vi "Run.vi"(8 "error in (no error)":errorcluster, 11 "Channel in":refnum<class "Channel.lvclass">) -> (0 "error out":errorcluster, 3 "Channel out":refnum<class "Channel.lvclass">)   [LabVIEW 2018, in "Channel.lvclass"]
doc: "Run the channel"
uses:
  Channel.lvclass
  Channel.lvclass/Channel.ctl
  Simulated_CCD_Camera/Simulated_CCD_Camera.lvclass/Simulated_CCD_Camera.ctl
  State Machine/State Machine.lvclass
  Simulated_CCD_Camera/Simulated_CCD_Camera.lvclass
  RxTx/RxTx.lvclass
  Header content/Header content.lvclass
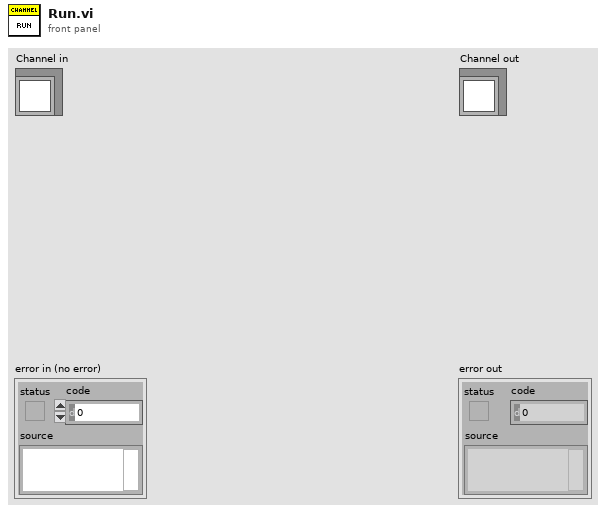
[diagram p1: front panel]
types:
  T1 = cluster{"PREAMP":u16, "READOUT_RATE":u16, "EM_GAIN":u16, "VERTICAL_SHIFT_SPEED":u16, "READ_MODE":u16, "FRAME_TRANSFER":bool, "VERTICAL_CLOCK_VOLTAGE":u16, "ACQUISITION_MODE":u16, "AD_CHANNEL":u16, "EM_MODE":u16, "SHUTTER_TTL":u16, "SHUTTER_OPENING_TIME":u16, "SHUTTER_CLOSING_TIME":u16, "SHUTTER_MODE":u16, "TRIGGER_MODE":u16, "VBIN":u16, "INITIAL_LINE":u16, "INITIAL_COLUMN":u16, "FINAL_LINE":u16, "FINAL_COLUMN":u16, "HBIN":u16}
  T2 = cluster{"CYCLES_DONE":u16, "LAST_IMAGE_NAME":string, "DISK_SPACE":u16, "FRAMES_DONE":u16, "CCD_STATUS":string, "CURRENT_TEMPERATURE":i16, "TEMPERATURE_STATUS":string, "FRAME_EXPOSURE_TIME":sgl, "ERROR":bool, "SERIAL_NUMBER":u16, "ACQUIRING":bool, "IMAGE_INDEX":u32, "SEQS_DONE":u16}
  T3 = cluster{"COOLER_POWER_STATUS":u16, "TEMP":i32, "EXPTIME":dbl, "#FRAMES":u32, "#CYCLES":u32, "COMMENT":string, "OBSTYPE":string, "OBJECT":string, "OBSERVER":string, "FILTER":string, "CTRLINTE":string, "INSTMODE":string, "#SEQS":u32, "WAVEPLATE_POS":u16, "TCSMODE":bool, "INSTROT":dbl, "ICSMODE":u8}
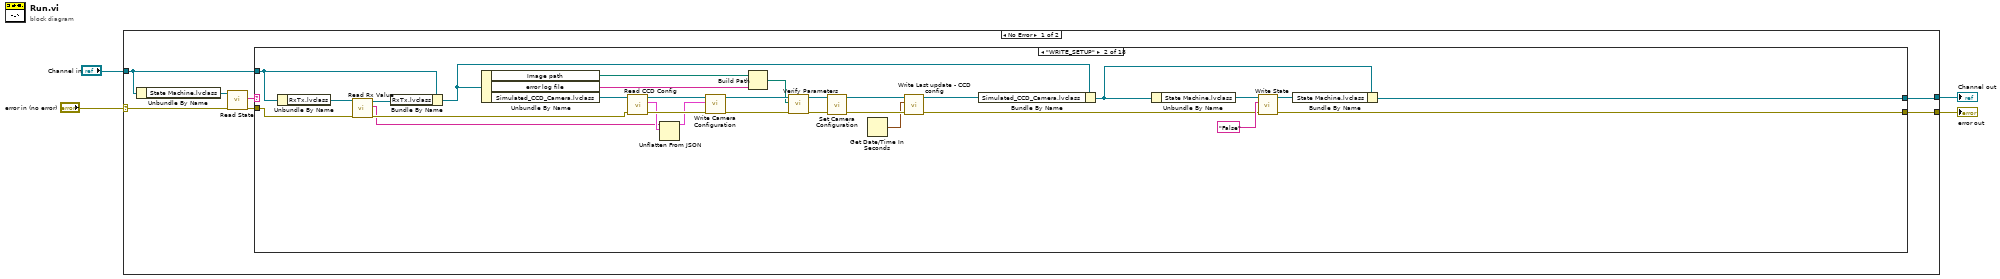
[diagram p0: block diagram]
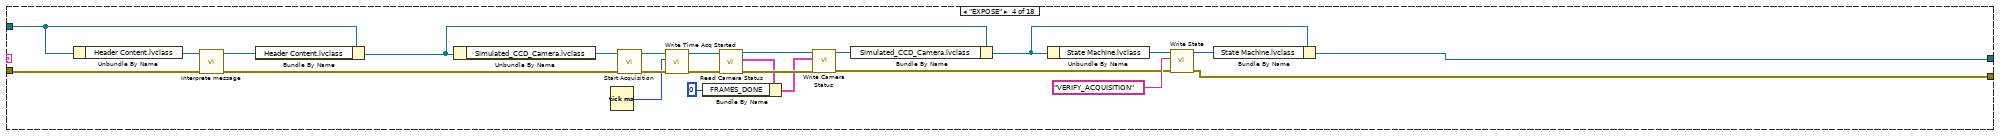
[diagram p4: hidden frame]
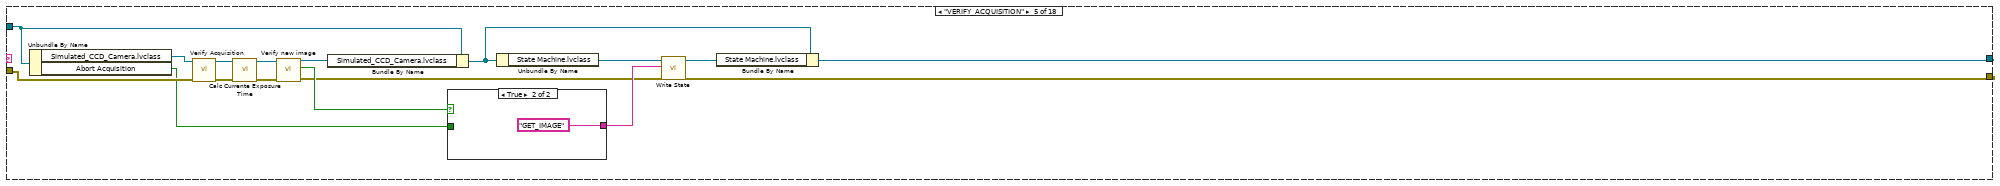
[diagram p5: hidden frame]
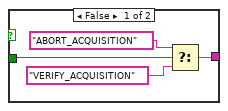
[diagram p6: hidden frame]
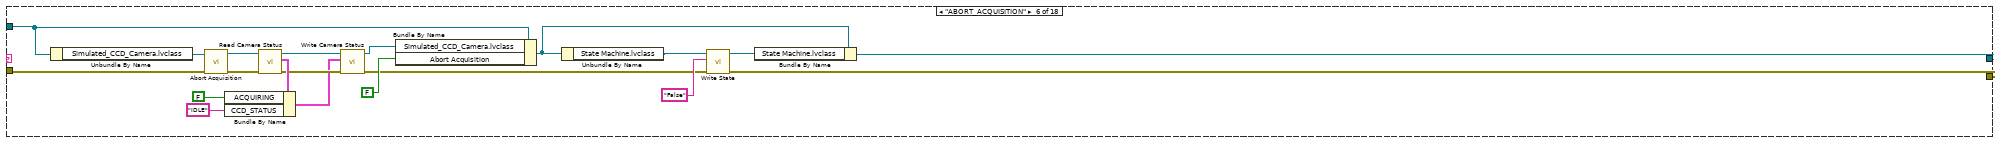
[diagram p7: hidden frame]
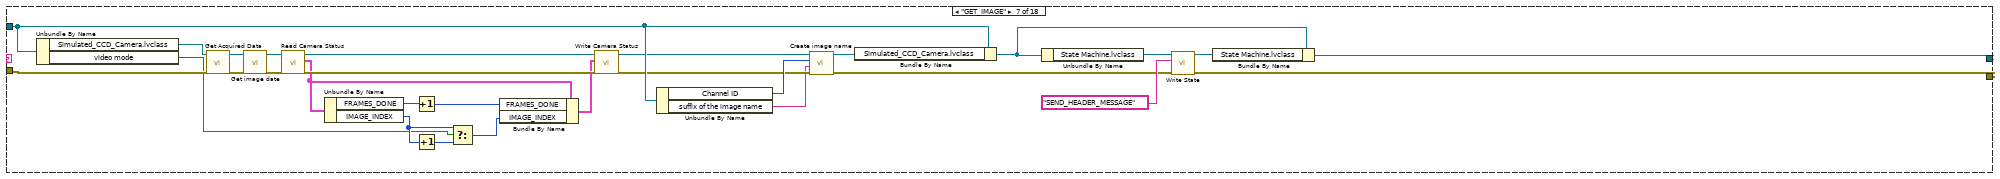
[diagram p8: hidden frame]
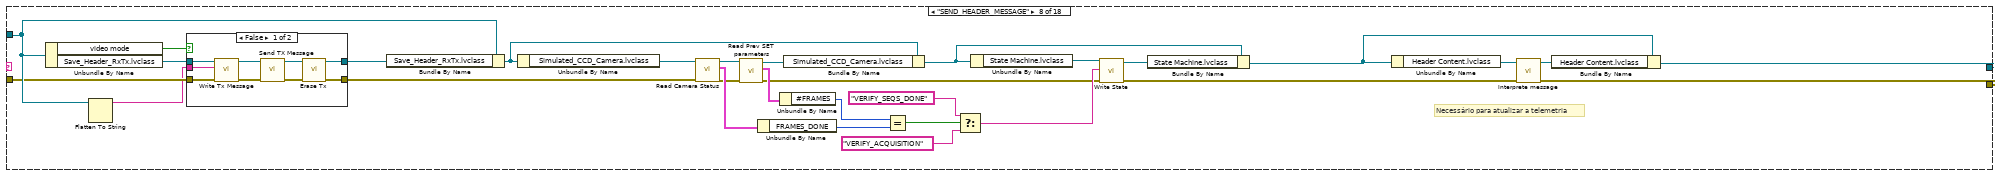
[diagram p9: hidden frame]
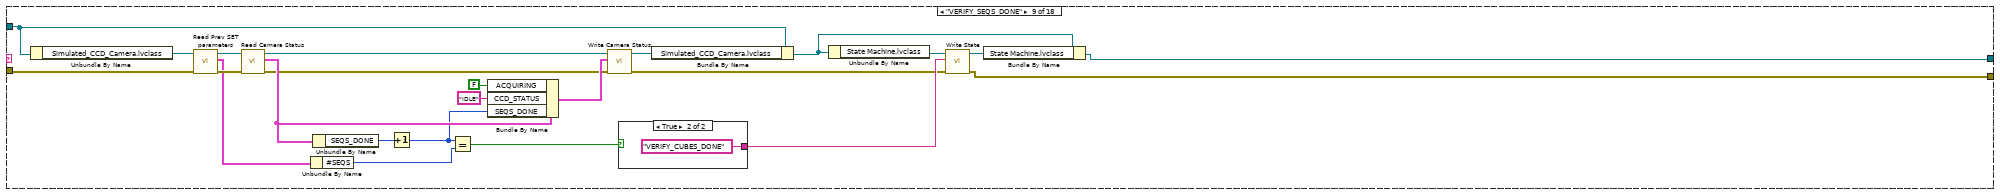
[diagram p11: hidden frame]
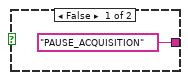
[diagram p12: hidden frame]
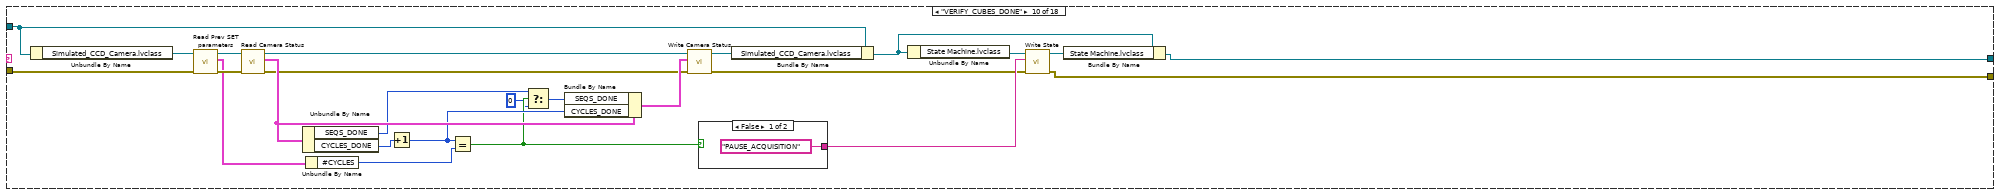
[diagram p13: hidden frame]
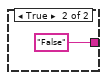
[diagram p14: hidden frame]
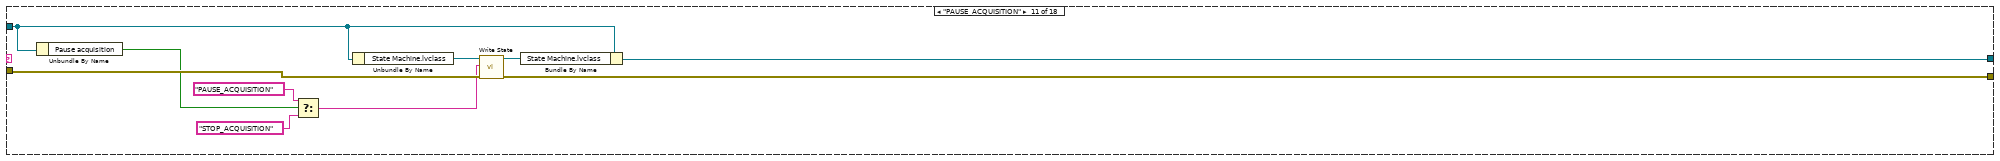
[diagram p15: hidden frame]
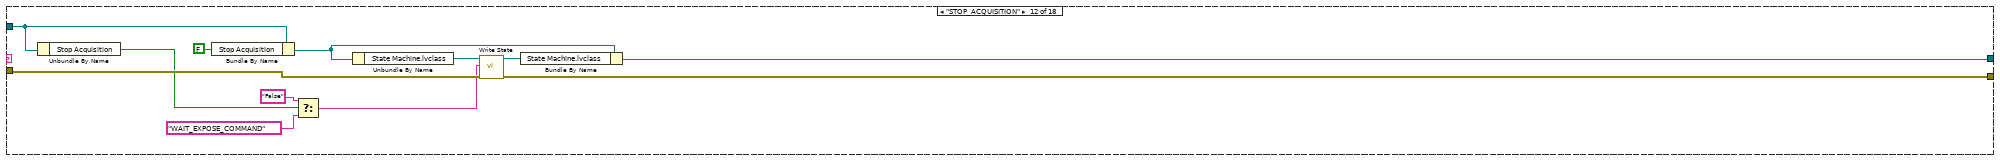
[diagram p16: hidden frame]
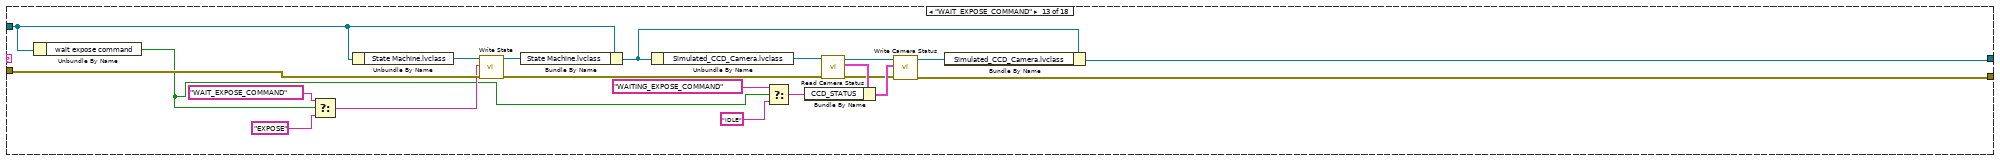
[diagram p17: hidden frame]
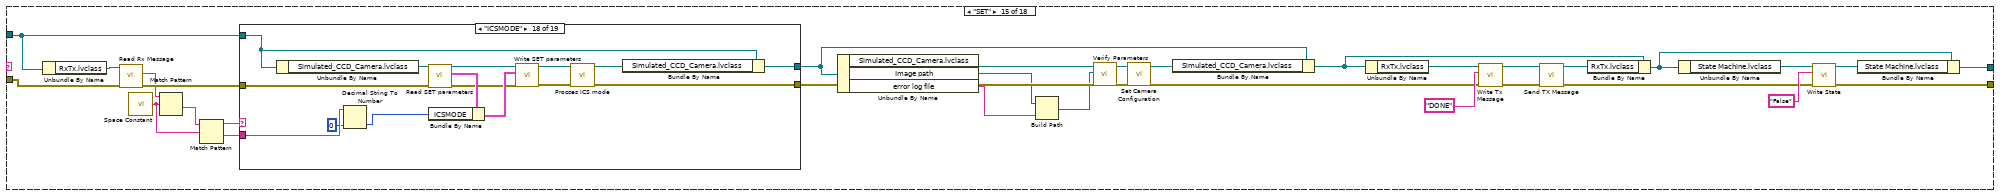
[diagram p19: hidden frame]
diagram:
  n1 = case shown="No Error" "error in (no error)" {
    selector: "error in (no error)" -> [w7 w618]
    tunnel: [w11 w618] -> w3
    tunnel: [w9 w617] -> w1
    tunnel: "Channel in" -> [w10 w617]
    frame No Error {
      n2 = Unbundle By Name(w10) -> ("State Machine.lvclass"=w8:refnum<class "State Machine.lvclass">)
      n3 = call-dynamic "Read State.vi"("error in (no error)"=w7, "State Machine in"=w8) -> ("error out"=w6:errorcluster, "State"=w5:string)  [unwired: 7 in, 1 out]
      n4 = case shown="\"WRITE_SETUP\"" w5 {
        tunnel: w6 -> [w12 w35 w44 w50 w75 w97 w136 w152 w193 w221 w243 w254 w276 w279 w302 w544 w604 w613]
        tunnel: [w12 w38 w44 w66 w82 w108 w138 w142 w187 w215 w241 w252 w262 w279 w304 w537 w595 w605] -> w11
        tunnel: [w13 w39 w45 w65 w85 w111 w119 w143 w188 w216 w240 w251 w263 w280 w305 w538 w602 w606] -> w9
        tunnel: w10 -> [w13 w42 w45 w49 w87 w96 w128 w154 w198 w228 w242 w253 w275 w280 w311 w535 w603 w610]
        frame "False", Default {
        }
        frame "WRITE_SETUP" {
          n5 = Unbundle By Name(w42) -> ("RxTx.lvclass"=w36:refnum<class "RxTx.lvclass">)
          n6 = call "Read Rx Value.vi"("error in (no error)"=w35, "RxTx in"=w36) -> ("error out"=w30:errorcluster, "Rx value"=w27:string, "RxTx out"=w34:refnum<class "RxTx.lvclass">)  [unwired: 7 in]
          n7 = Bundle By Name(cluster=w42, "RxTx.lvclass"=w34) -> (w43:refnum<class "Channel.lvclass">)
          n8 = Unbundle By Name(w43) -> ("Image path"=w14:path, "error log file"=w15:string, "Simulated_CCD_Camera.lvclass"=w33:refnum<class "Simulated_CCD_Camera.lvclass">)
          n9 = call "Read CCD Config.vi"("error in (no error)"=w30, "CCDCamera in"=w33) -> ("error out"=w31:errorcluster, "CCD Config"=w29:T1, "CCDCamera out"=w32:refnum<class "Simulated_CCD_Camera.lvclass">)  [unwired: 7 in]
          n10 = Unflatten From JSON(JSON string=w27, type and defaults=w29) -> (value=w28:T1)  [unwired: 5 in, 1 out]
          n11 = call-dynamic "Write Camera Configuration.vi"("error in (no error)"=w31, "CCD Config"=w28, "CCDCamera in"=w32) -> ("error out"=w25:errorcluster, "CCDCamera out"=w24:refnum<class "Simulated_CCD_Camera.lvclass">)  [unwired: 7 in]
          n12 = Build Path(base path=w14, name or relative path=w15) -> (appended path=w16:path)
          n13 = call "Verify Parameters.vi"("error in (no error)"=w25, "error file"=w16, "Simulated_CCD_Camera in"=w24) -> ("error out"=w23:errorcluster, "Simulated_CCD_Camera out"=w22:refnum<class "Simulated_CCD_Camera.lvclass">)  [unwired: 7 in]
          n14 = call-dynamic "Set Camera Configuration.vi"("error in (no error)"=w23, "CCDCamera in"=w22) -> ("error out"=w19:errorcluster, "CCDCamera out"=w21:refnum<class "Simulated_CCD_Camera.lvclass">)  [unwired: 8 in]
          n15 = Get Date/Time In Seconds() -> (seconds since 1Jan1904=w17:timestamp)
          n16 = call-dynamic "Write Last update - CCD config.vi"("error in (no error)"=w19, "Last update - CCD config"=w17, "Simulated_CCD_Camera in"=w21) -> ("error out"=w18:errorcluster, "Simulated_CCD_Camera out"=w20:refnum<class "Simulated_CCD_Camera.lvclass">)  [unwired: 7 in]
          n17 = Bundle By Name(cluster=w43, "Simulated_CCD_Camera.lvclass"=w20) -> (w37:refnum<class "Channel.lvclass">)
          n18 = Unbundle By Name(w37) -> ("State Machine.lvclass"=w40:refnum<class "State Machine.lvclass">)
          n19 = call-dynamic "Write State.vi"("error in (no error)"=w18, "State"="False", "State Machine in"=w40) -> ("error out"=w38:errorcluster, "State Machine out"=w41:refnum<class "State Machine.lvclass">)  [unwired: 7 in]
          n20 = Bundle By Name(cluster=w37, "State Machine.lvclass"=w41) -> (w39:refnum<class "Channel.lvclass">)
        }
        frame "---------------------------------" {
        }
        frame "EXPOSE" {
          n21 = Unbundle By Name(w49) -> ("Header Content.lvclass"=w51:refnum<class "Header content.lvclass">)
          n22 = call "Interprete message.vi"("error in (no error)"=w50, "TCS_ACS in"=w51) -> ("error out"=w47:errorcluster, "TCS_ACS out"=w48:refnum<class "Header content.lvclass">)  [unwired: 8 in]
          n23 = Bundle By Name(cluster=w49, "Header Content.lvclass"=w48) -> (w46:refnum<class "Channel.lvclass">)
          n24 = Unbundle By Name(w46) -> ("Simulated_CCD_Camera.lvclass"=w68:refnum<class "Simulated_CCD_Camera.lvclass">)
          n25 = Tick Count (ms)() -> (millisecond timer value=w61:u32)
          n26 = call-dynamic "Start Acquisition.vi"("error in (no error)"=w47, "CCDCamera in"=w68) -> ("error out"=w62:errorcluster, "CCDCamera out"=w63:refnum<class "Simulated_CCD_Camera.lvclass">)  [unwired: 8 in]
          n27 = call "Write Time Acq Started.vi"("error in (no error)"=w62, "Time Acq Started"=w61, "Simulated_CCD_Camera in"=w63) -> ("error out"=w57:errorcluster, "Simulated_CCD_Camera out"=w58:refnum<class "Simulated_CCD_Camera.lvclass">)  [unwired: 7 in]
          n28 = call "Read Camera Status.vi"("error in (no error)"=w57, "CCDCamera in"=w58) -> ("error out"=w56:errorcluster, "Camera Status"=w54:T2, "CCDCamera out"=w55:refnum<class "Simulated_CCD_Camera.lvclass">)  [unwired: 7 in]
          n29 = Bundle By Name(cluster=w54, "FRAMES_DONE"=u16 0) -> (w53:T2)
          n30 = call "Write Camera Status.vi"("error in (no error)"=w56, "Camera Status"=w53, "CCDCamera in"=w55) -> ("error out"=w59:errorcluster, "CCDCamera out"=w60:refnum<class "Simulated_CCD_Camera.lvclass">)  [unwired: 7 in]
          n31 = Bundle By Name(cluster=w46, "Simulated_CCD_Camera.lvclass"=w60) -> (w64:refnum<class "Channel.lvclass">)
          n32 = Unbundle By Name(w64) -> ("State Machine.lvclass"=w70:refnum<class "State Machine.lvclass">)
          n33 = call-dynamic "Write State.vi"("error in (no error)"=w59, "State"="VERIFY_ACQUISITION", "State Machine in"=w70) -> ("error out"=w66:errorcluster, "State Machine out"=w67:refnum<class "State Machine.lvclass">)  [unwired: 7 in]
          n34 = Bundle By Name(cluster=w64, "State Machine.lvclass"=w67) -> (w65:refnum<class "Channel.lvclass">)
        }
        frame "VERIFY_ACQUISITION" {
          n35 = Unbundle By Name(w87) -> ("Simulated_CCD_Camera.lvclass"=w76:refnum<class "Simulated_CCD_Camera.lvclass">, "Abort Acquisition"=w74:bool)
          n36 = call-dynamic "Verify Acquisition.vi"("error in (no error)"=w75, "CCDCamera in"=w76) -> ("error out"=w78:errorcluster, "CCDCamera out"=w73:refnum<class "Simulated_CCD_Camera.lvclass">)  [unwired: 8 in]
          n37 = call-dynamic "Calc Currente Exposure Time.vi"("error in (no error)"=w78, "CCDCamera in"=w73) -> ("error out"=w79:errorcluster, "CCDCamera out"=w71:refnum<class "Simulated_CCD_Camera.lvclass">)  [unwired: 8 in]
          n38 = call-dynamic "Verify new image.vi"("error in (no error)"=w79, "CCDCamera in"=w71) -> ("error out"=w77:errorcluster, "New Images ?"=w80:bool, "CCDCamera out"=w72:refnum<class "Simulated_CCD_Camera.lvclass">)  [unwired: 7 in]
          n39 = Bundle By Name(cluster=w87, "Simulated_CCD_Camera.lvclass"=w72) -> (w86:refnum<class "Channel.lvclass">)
          n40 = case shown="True" w80 {
            tunnel: [w89 "GET_IMAGE"] -> w81
            tunnel: w74 -> [w88 _]
            frame False {
              n41 = Select(t="ABORT_ACQUISITION", s=w88, f="VERIFY_ACQUISITION") -> (s? t:f=w89:string)
            }
            frame True {
            }
          }
          n42 = Unbundle By Name(w86) -> ("State Machine.lvclass"=w84:refnum<class "State Machine.lvclass">)
          n43 = call-dynamic "Write State.vi"("error in (no error)"=w77, "State"=w81, "State Machine in"=w84) -> ("error out"=w82:errorcluster, "State Machine out"=w83:refnum<class "State Machine.lvclass">)  [unwired: 7 in]
          n44 = Bundle By Name(cluster=w86, "State Machine.lvclass"=w83) -> (w85:refnum<class "Channel.lvclass">)
        }
        frame "ABORT_ACQUISITION" {
          n45 = Unbundle By Name(w96) -> ("Simulated_CCD_Camera.lvclass"=w98:refnum<class "Simulated_CCD_Camera.lvclass">)
          n46 = call-dynamic "Abort Acquisition.vi"("error in (no error)"=w97, "CCDCamera in"=w98) -> ("error out"=w103:errorcluster, "CCDCamera out"=w104:refnum<class "Simulated_CCD_Camera.lvclass">)  [unwired: 8 in]
          n47 = call "Read Camera Status.vi"("error in (no error)"=w103, "CCDCamera in"=w104) -> ("error out"=w101:errorcluster, "Camera Status"=w106:T2, "CCDCamera out"=w102:refnum<class "Simulated_CCD_Camera.lvclass">)  [unwired: 7 in]
          n48 = Bundle By Name(cluster=w106, "ACQUIRING"=FALSE ("Acquiring"), "CCD_STATUS"="IDLE" ("STATUS")) -> (w100:T2)
          n49 = call "Write Camera Status.vi"("error in (no error)"=w101, "Camera Status"=w100, "CCDCamera in"=w102) -> ("error out"=w94:errorcluster, "CCDCamera out"=w93:refnum<class "Simulated_CCD_Camera.lvclass">)  [unwired: 7 in]
          n50 = Bundle By Name(cluster=w96, "Simulated_CCD_Camera.lvclass"=w93, "Abort Acquisition"=FALSE ("Acquiring")) -> (w112:refnum<class "Channel.lvclass">)
          n51 = Unbundle By Name(w112) -> ("State Machine.lvclass"=w110:refnum<class "State Machine.lvclass">)
          n52 = call-dynamic "Write State.vi"("error in (no error)"=w94, "State"="False", "State Machine in"=w110) -> ("error out"=w108:errorcluster, "State Machine out"=w109:refnum<class "State Machine.lvclass">)  [unwired: 7 in]
          n53 = Bundle By Name(cluster=w112, "State Machine.lvclass"=w109) -> (w111:refnum<class "Channel.lvclass">)
        }
        frame "GET_IMAGE" {
          n54 = Unbundle By Name(w128) -> ("Simulated_CCD_Camera.lvclass"=w116:refnum<class "Simulated_CCD_Camera.lvclass">, "video mode"=w113:bool)
          n55 = call-dynamic "Get Acquired Data.vi"("error in (no error)"=w136, "CCDCamera in"=w116) -> ("error out"=w120:errorcluster, "CCDCamera out"=w123:refnum<class "Simulated_CCD_Camera.lvclass">)  [unwired: 8 in]
          n56 = call-dynamic "Get image date.vi"("error in (no error)"=w120, "Simulated_CCD_Camera in"=w123) -> ("error out"=w121:errorcluster, "Simulated_CCD_Camera out"=w122:refnum<class "Simulated_CCD_Camera.lvclass">)  [unwired: 8 in]
          n57 = call "Read Camera Status.vi"("error in (no error)"=w121, "CCDCamera in"=w122) -> ("error out"=w135:errorcluster, "Camera Status"=w131:T2, "CCDCamera out"=w134:refnum<class "Simulated_CCD_Camera.lvclass">)  [unwired: 7 in]
          n58 = Unbundle By Name(w131) -> ("FRAMES_DONE"=w133:u16, "IMAGE_INDEX"=w114:u32)
          n59 = Increment(x=w133) -> (x+1=w117:u16)
          n60 = Increment(x=w114) -> (x+1=w115:u32)
          n61 = Select(t=w114, s=w113, f=w115) -> (s? t:f=w118:u32)
          n62 = Bundle By Name(cluster=w131, "FRAMES_DONE"=w117, "IMAGE_INDEX"=w118) -> (w132:T2)
          n63 = call "Write Camera Status.vi"("error in (no error)"=w135, "Camera Status"=w132, "CCDCamera in"=w134) -> ("error out"=w125:errorcluster, "CCDCamera out"=w126:refnum<class "Simulated_CCD_Camera.lvclass">)  [unwired: 7 in]
          n64 = Unbundle By Name(w128) -> ("Channel ID"=w127:u8, "suffix of the image name"=w124:string)
          n65 = call "Create image name.vi"("error in (no error)"=w125, "Suffix"=w124, "Channel"=w127, "Simulated_CCD_Camera in"=w126) -> ("error out"=w129:errorcluster, "Simulated_CCD_Camera out"=w130:refnum<class "Simulated_CCD_Camera.lvclass">)  [unwired: 6 in]
          n66 = Bundle By Name(cluster=w128, "Simulated_CCD_Camera.lvclass"=w130) -> (w141:refnum<class "Channel.lvclass">)
          n67 = Unbundle By Name(w141) -> ("State Machine.lvclass"=w139:refnum<class "State Machine.lvclass">)
          n68 = call-dynamic "Write State.vi"("error in (no error)"=w129, "State"="SEND_HEADER_MESSAGE", "State Machine in"=w139) -> ("error out"=w138:errorcluster, "State Machine out"=w140:refnum<class "State Machine.lvclass">)  [unwired: 7 in]
          n69 = Bundle By Name(cluster=w141, "State Machine.lvclass"=w140) -> (w119:refnum<class "Channel.lvclass">)
        }
        frame "SEND_HEADER_MESSAGE" {
          # "Necessário para atualizar a telemetria"
          n70 = Unbundle By Name(w154) -> ("video mode"=w148:bool, "Save_Header_RxTx.lvclass"=w153:refnum<class "RxTx.lvclass">)
          n71 = Flatten To String(anything=w154) -> (data string=w149:string)  [unwired: 3 in, 2 out]
          n72 = case shown="False" w148 {
            tunnel: w153 -> [w180 w182]
            tunnel: w152 -> [w177 w181]
            tunnel: [w175 w182] -> w151
            tunnel: [w173 w181] -> w150
            tunnel: w149 -> [w172 _]
            frame False {
              n73 = call "Write Tx Message.vi"("error in (no error)"=w177, "Tx Message"=w172, "RxTx in"=w180) -> ("error out"=w178:errorcluster, "RxTx out"=w179:refnum<class "RxTx.lvclass">)  [unwired: 7 in]
              n74 = call "Send TX Message.vi"("error in (no error)"=w178, "RxTx in"=w179) -> ("error out"=w174:errorcluster, "RxTx out"=w176:refnum<class "RxTx.lvclass">)  [unwired: 8 in]
              n75 = call "Erase Tx.vi"("error in (no error)"=w174, "RxTx in"=w176) -> ("error out"=w173:errorcluster, "RxTx out"=w175:refnum<class "RxTx.lvclass">)  [unwired: 8 in]
            }
            frame True {
            }
          }
          n76 = Bundle By Name(cluster=w154, "Save_Header_RxTx.lvclass"=w151) -> (w167:refnum<class "Channel.lvclass">)
          n77 = Unbundle By Name(w167) -> ("Simulated_CCD_Camera.lvclass"=w162:refnum<class "Simulated_CCD_Camera.lvclass">)
          n78 = call "Read Camera Status.vi"("error in (no error)"=w150, "CCDCamera in"=w162) -> ("error out"=w158:errorcluster, "Camera Status"=w161:T2, "CCDCamera out"=w160:refnum<class "Simulated_CCD_Camera.lvclass">)  [unwired: 7 in]
          n79 = call-dynamic "Read Prev SET parameters.vi"("error in (no error)"=w158, "Simulated_CCD_Camera in"=w160) -> ("error out"=w155:errorcluster, "Old SET parameters"=w157:T3, "Simulated_CCD_Camera out"=w159:refnum<class "Simulated_CCD_Camera.lvclass">)  [unwired: 7 in]
          n80 = Unbundle By Name(w161) -> ("FRAMES_DONE"=w169:u16)
          n81 = Unbundle By Name(w157) -> ("#FRAMES"=w156:u32)
          n82 = Bundle By Name(cluster=w167, "Simulated_CCD_Camera.lvclass"=w159) -> (w165:refnum<class "Channel.lvclass">)
          n83 = Equal?(x=w156, y=w169) -> (x = y?=w168:bool)
          n84 = Select(t="VERIFY_SEQS_DONE", s=w168, f="VERIFY_ACQUISITION") -> (s? t:f=w166:string)
          n85 = Unbundle By Name(w165) -> ("State Machine.lvclass"=w170:refnum<class "State Machine.lvclass">)
          n86 = call-dynamic "Write State.vi"("error in (no error)"=w155, "State"=w166, "State Machine in"=w170) -> ("error out"=w144:errorcluster, "State Machine out"=w171:refnum<class "State Machine.lvclass">)  [unwired: 7 in]
          n87 = Bundle By Name(cluster=w165, "State Machine.lvclass"=w171) -> (w145:refnum<class "Channel.lvclass">)
          n88 = Unbundle By Name(w145) -> ("Header Content.lvclass"=w147:refnum<class "Header content.lvclass">)
          n89 = call "Interprete message.vi"("error in (no error)"=w144, "TCS_ACS in"=w147) -> ("error out"=w142:errorcluster, "TCS_ACS out"=w146:refnum<class "Header content.lvclass">)  [unwired: 8 in]
          n90 = Bundle By Name(cluster=w145, "Header Content.lvclass"=w146) -> (w143:refnum<class "Channel.lvclass">)
        }
        frame "VERIFY_SEQS_DONE" {
          n91 = Unbundle By Name(w198) -> ("Simulated_CCD_Camera.lvclass"=w196:refnum<class "Simulated_CCD_Camera.lvclass">)
          n92 = call-dynamic "Read Prev SET parameters.vi"("error in (no error)"=w193, "Simulated_CCD_Camera in"=w196) -> ("error out"=w194:errorcluster, "Old SET parameters"=w192:T3, "Simulated_CCD_Camera out"=w195:refnum<class "Simulated_CCD_Camera.lvclass">)  [unwired: 7 in]
          n93 = call "Read Camera Status.vi"("error in (no error)"=w194, "CCDCamera in"=w195) -> ("error out"=w185:errorcluster, "Camera Status"=w204:T2, "CCDCamera out"=w186:refnum<class "Simulated_CCD_Camera.lvclass">)  [unwired: 7 in]
          n94 = Unbundle By Name(w192) -> ("#SEQS"=w191:u32)
          n95 = Unbundle By Name(w204) -> ("SEQS_DONE"=w203:u16)
          n96 = Increment(x=w203) -> (x+1=w201:u16)
          n97 = Equal?(x=w201, y=w191) -> (x = y?=w199:bool)
          n98 = Bundle By Name(cluster=w204, "ACQUIRING"=FALSE, "CCD_STATUS"="IDLE", "SEQS_DONE"=w201) -> (w202:T2)
          n99 = call "Write Camera Status.vi"("error in (no error)"=w185, "Camera Status"=w202, "CCDCamera in"=w186) -> ("error out"=w189:errorcluster, "CCDCamera out"=w190:refnum<class "Simulated_CCD_Camera.lvclass">)  [unwired: 7 in]
          n100 = case shown="True" w199 {
            tunnel: ["PAUSE_ACQUISITION" "VERIFY_CUBES_DONE"] -> w205
            frame False {
            }
            frame True {
            }
          }
          n101 = Bundle By Name(cluster=w198, "Simulated_CCD_Camera.lvclass"=w190) -> (w197:refnum<class "Channel.lvclass">)
          n102 = Unbundle By Name(w197) -> ("State Machine.lvclass"=w200:refnum<class "State Machine.lvclass">)
          n103 = call-dynamic "Write State.vi"("error in (no error)"=w189, "State"=w205, "State Machine in"=w200) -> ("error out"=w187:errorcluster, "State Machine out"=w206:refnum<class "State Machine.lvclass">)  [unwired: 7 in]
          n104 = Bundle By Name(cluster=w197, "State Machine.lvclass"=w206) -> (w188:refnum<class "Channel.lvclass">)
        }
        frame "VERIFY_CUBES_DONE" {
          n105 = Unbundle By Name(w228) -> ("Simulated_CCD_Camera.lvclass"=w224:refnum<class "Simulated_CCD_Camera.lvclass">)
          n106 = call-dynamic "Read Prev SET parameters.vi"("error in (no error)"=w221, "Simulated_CCD_Camera in"=w224) -> ("error out"=w222:errorcluster, "Old SET parameters"=w220:T3, "Simulated_CCD_Camera out"=w223:refnum<class "Simulated_CCD_Camera.lvclass">)  [unwired: 7 in]
          n107 = call "Read Camera Status.vi"("error in (no error)"=w222, "CCDCamera in"=w223) -> ("error out"=w225:errorcluster, "Camera Status"=w231:T2, "CCDCamera out"=w226:refnum<class "Simulated_CCD_Camera.lvclass">)  [unwired: 7 in]
          n108 = Unbundle By Name(w231) -> ("SEQS_DONE"=w210:u16, "CYCLES_DONE"=w209:u16)
          n109 = Unbundle By Name(w220) -> ("#CYCLES"=w219:u32)
          n110 = Increment(x=w209) -> (x+1=w214:u16)
          n111 = Equal?(x=w214, y=w219) -> (x = y?=w212:bool)
          n112 = Select(t=w210, s=w212, f=0) -> (s? t:f=w213:i32)
          n113 = Bundle By Name(cluster=w231, "SEQS_DONE"=w213, "CYCLES_DONE"=w214) -> (w230:T2)
          n114 = call "Write Camera Status.vi"("error in (no error)"=w225, "Camera Status"=w230, "CCDCamera in"=w226) -> ("error out"=w217:errorcluster, "CCDCamera out"=w218:refnum<class "Simulated_CCD_Camera.lvclass">)  [unwired: 7 in]
          n115 = case shown="False" w212 {
            tunnel: ["PAUSE_ACQUISITION" "False"] -> w232
            frame False {
            }
            frame True {
            }
          }
          n116 = Bundle By Name(cluster=w228, "Simulated_CCD_Camera.lvclass"=w218) -> (w227:refnum<class "Channel.lvclass">)
          n117 = Unbundle By Name(w227) -> ("State Machine.lvclass"=w229:refnum<class "State Machine.lvclass">)
          n118 = call-dynamic "Write State.vi"("error in (no error)"=w217, "State"=w232, "State Machine in"=w229) -> ("error out"=w215:errorcluster, "State Machine out"=w233:refnum<class "State Machine.lvclass">)  [unwired: 7 in]
          n119 = Bundle By Name(cluster=w227, "State Machine.lvclass"=w233) -> (w216:refnum<class "Channel.lvclass">)
        }
        frame "PAUSE_ACQUISITION" {
          n120 = Unbundle By Name(w242) -> ("Pause acquisition"=w238:bool)
          n121 = Select(t="PAUSE_ACQUISITION", s=w238, f="STOP_ACQUISITION") -> (s? t:f=w239:string)
          n122 = Unbundle By Name(w242) -> ("State Machine.lvclass"=w245:refnum<class "State Machine.lvclass">)
          n123 = call-dynamic "Write State.vi"("error in (no error)"=w243, "State"=w239, "State Machine in"=w245) -> ("error out"=w241:errorcluster, "State Machine out"=w244:refnum<class "State Machine.lvclass">)  [unwired: 7 in]
          n124 = Bundle By Name(cluster=w242, "State Machine.lvclass"=w244) -> (w240:refnum<class "Channel.lvclass">)
        }
        frame "STOP_ACQUISITION" {
          n125 = Unbundle By Name(w253) -> ("Stop Acquisition"=w246:bool)
          n126 = Bundle By Name(cluster=w253, "Stop Acquisition"=FALSE) -> (w255:refnum<class "Channel.lvclass">)
          n127 = Select(t="False", s=w246, f="WAIT_EXPOSE_COMMAND") -> (s? t:f=w248:string)
          n128 = Unbundle By Name(w255) -> ("State Machine.lvclass"=w257:refnum<class "State Machine.lvclass">)
          n129 = call-dynamic "Write State.vi"("error in (no error)"=w254, "State"=w248, "State Machine in"=w257) -> ("error out"=w252:errorcluster, "State Machine out"=w256:refnum<class "State Machine.lvclass">)  [unwired: 7 in]
          n130 = Bundle By Name(cluster=w255, "State Machine.lvclass"=w256) -> (w251:refnum<class "Channel.lvclass">)
        }
        frame "WAIT_EXPOSE_COMMAND" {
          n131 = Unbundle By Name(w275) -> ("wait expose command"=w258:bool)
          n132 = Select(t="WAIT_EXPOSE_COMMAND", s=w258, f="EXPOSE") -> (s? t:f=w272:string)
          n133 = Unbundle By Name(w275) -> ("State Machine.lvclass"=w278:refnum<class "State Machine.lvclass">)
          n134 = call-dynamic "Write State.vi"("error in (no error)"=w276, "State"=w272, "State Machine in"=w278) -> ("error out"=w270:errorcluster, "State Machine out"=w277:refnum<class "State Machine.lvclass">)  [unwired: 7 in]
          n135 = Bundle By Name(cluster=w275, "State Machine.lvclass"=w277) -> (w265:refnum<class "Channel.lvclass">)
          n136 = Unbundle By Name(w265) -> ("Simulated_CCD_Camera.lvclass"=w271:refnum<class "Simulated_CCD_Camera.lvclass">)
          n137 = Select(t="WAITING_EXPOSE_COMMAND" ("CCD_STATUS"), s=w258, f="IDLE" ("CCD_STATUS")) -> (s? t:f=w260:string)
          n138 = call "Read Camera Status.vi"("error in (no error)"=w270, "CCDCamera in"=w271) -> ("error out"=w267:errorcluster, "Camera Status"=w269:T2, "CCDCamera out"=w266:refnum<class "Simulated_CCD_Camera.lvclass">)  [unwired: 7 in]
          n139 = Bundle By Name(cluster=w269, "CCD_STATUS"=w260) -> (w268:T2)
          n140 = call "Write Camera Status.vi"("error in (no error)"=w267, "Camera Status"=w268, "CCDCamera in"=w266) -> ("error out"=w262:errorcluster, "CCDCamera out"=w264:refnum<class "Simulated_CCD_Camera.lvclass">)  [unwired: 7 in]
          n141 = Bundle By Name(cluster=w265, "Simulated_CCD_Camera.lvclass"=w264) -> (w263:refnum<class "Channel.lvclass">)
        }
        frame "------------------------------" {
        }
        frame "SET" {
          n142 = Unbundle By Name(w311) -> ("RxTx.lvclass"=w301:refnum<class "RxTx.lvclass">)
          n143 = call "Read Rx Message.vi"("error in (no error)"=w302, "RxTx in"=w301) -> ("error out"=w303:errorcluster, "Rx Message"=w299:string)  [unwired: 7 in, 1 out]
          n144 = call <vilib>:"Space Constant.vi"() -> ("String"=w298:string)
          n145 = Match Pattern(string=w299, regular expression=w298) -> (after substring=w300:string)  [unwired: 1 in, 3 out]
          n146 = Match Pattern(string=w300, regular expression=w298) -> (before substring=w297:string, after substring=w296:string)  [unwired: 1 in, 2 out]
          n147 = case shown="\"ICSMODE\"" w297 {
            tunnel: [w314 w326 w339 w352 w365 w378 w392 w405 w418 w429 w440 w451 w462 w473 w484 w495 w508 w523 w528] -> w291
            tunnel: w311 -> [w314 w327 w340 w353 w366 w379 w393 w406 w419 w430 w441 w452 w463 w474 w485 w496 w509 w524 w529]
            tunnel: [w313 w319 w332 w345 w358 w371 w380 w398 w411 w425 w436 w447 w458 w469 w480 w491 w504 w510 w527] -> w292
            tunnel: w303 -> [w313 w321 w334 w347 w360 w373 w390 w400 w413 w427 w438 w449 w460 w471 w482 w493 w506 w521 w527]
            tunnel: w296 -> [_ w323 w336 w349 w362 w375 w384 w402 w415 w420 w431 w442 w453 w464 w475 w486 w498 w516 w525]
            frame "False", Default {
            }
            frame "EXPTIME" {
              n148 = Unbundle By Name(w327) -> ("Simulated_CCD_Camera.lvclass"=w322:refnum<class "Simulated_CCD_Camera.lvclass">)
              n149 = Fract/Exp String To Number(string=w323, default (0 dbl)=0.0) -> (number=w324:dbl)  [unwired: 2 in, 1 out]
              n150 = call-dynamic "Read SET parameters.vi"("error in (no error)"=w321, "Simulated_CCD_Camera in"=w322) -> ("error out"=w315:errorcluster, "New SET parameters"=w318:T3, "Simulated_CCD_Camera out"=w316:refnum<class "Simulated_CCD_Camera.lvclass">)  [unwired: 7 in]
              n151 = Bundle By Name(cluster=w318, "EXPTIME"=w324) -> (w317:T3)
              n152 = call-dynamic "Write SET parameters.vi"("error in (no error)"=w315, "New SET parameters"=w317, "Simulated_CCD_Camera in"=w316) -> ("error out"=w319:errorcluster, "Simulated_CCD_Camera out"=w320:refnum<class "Simulated_CCD_Camera.lvclass">)  [unwired: 7 in]
              n153 = Bundle By Name(cluster=w327, "Simulated_CCD_Camera.lvclass"=w320) -> (w326:refnum<class "Channel.lvclass">)
            }
            frame "INSTROT" {
              n154 = Unbundle By Name(w340) -> ("Simulated_CCD_Camera.lvclass"=w335:refnum<class "Simulated_CCD_Camera.lvclass">)
              n155 = Fract/Exp String To Number(string=w336, default (0 dbl)=0.0) -> (number=w337:dbl)  [unwired: 2 in, 1 out]
              n156 = call-dynamic "Read SET parameters.vi"("error in (no error)"=w334, "Simulated_CCD_Camera in"=w335) -> ("error out"=w328:errorcluster, "New SET parameters"=w331:T3, "Simulated_CCD_Camera out"=w329:refnum<class "Simulated_CCD_Camera.lvclass">)  [unwired: 7 in]
              n157 = Bundle By Name(cluster=w331, "INSTROT"=w337) -> (w330:T3)
              n158 = call-dynamic "Write SET parameters.vi"("error in (no error)"=w328, "New SET parameters"=w330, "Simulated_CCD_Camera in"=w329) -> ("error out"=w332:errorcluster, "Simulated_CCD_Camera out"=w333:refnum<class "Simulated_CCD_Camera.lvclass">)  [unwired: 7 in]
              n159 = Bundle By Name(cluster=w340, "Simulated_CCD_Camera.lvclass"=w333) -> (w339:refnum<class "Channel.lvclass">)
            }
            frame "#FRAMES" {
              n160 = Unbundle By Name(w353) -> ("Simulated_CCD_Camera.lvclass"=w348:refnum<class "Simulated_CCD_Camera.lvclass">)
              n161 = Fract/Exp String To Number(string=w349, default (0 dbl)=u32 0) -> (number=w350:u32)  [unwired: 2 in, 1 out]
              n162 = call-dynamic "Read SET parameters.vi"("error in (no error)"=w347, "Simulated_CCD_Camera in"=w348) -> ("error out"=w341:errorcluster, "New SET parameters"=w344:T3, "Simulated_CCD_Camera out"=w342:refnum<class "Simulated_CCD_Camera.lvclass">)  [unwired: 7 in]
              n163 = Bundle By Name(cluster=w344, "#FRAMES"=w350) -> (w343:T3)
              n164 = call-dynamic "Write SET parameters.vi"("error in (no error)"=w341, "New SET parameters"=w343, "Simulated_CCD_Camera in"=w342) -> ("error out"=w345:errorcluster, "Simulated_CCD_Camera out"=w346:refnum<class "Simulated_CCD_Camera.lvclass">)  [unwired: 7 in]
              n165 = Bundle By Name(cluster=w353, "Simulated_CCD_Camera.lvclass"=w346) -> (w352:refnum<class "Channel.lvclass">)
            }
            frame "#CYCLES" {
              n166 = Unbundle By Name(w366) -> ("Simulated_CCD_Camera.lvclass"=w361:refnum<class "Simulated_CCD_Camera.lvclass">)
              n167 = Fract/Exp String To Number(string=w362, default (0 dbl)=u32 0) -> (number=w363:u32)  [unwired: 2 in, 1 out]
              n168 = call-dynamic "Read SET parameters.vi"("error in (no error)"=w360, "Simulated_CCD_Camera in"=w361) -> ("error out"=w354:errorcluster, "New SET parameters"=w357:T3, "Simulated_CCD_Camera out"=w355:refnum<class "Simulated_CCD_Camera.lvclass">)  [unwired: 7 in]
              n169 = Bundle By Name(cluster=w357, "#CYCLES"=w363) -> (w356:T3)
              n170 = call-dynamic "Write SET parameters.vi"("error in (no error)"=w354, "New SET parameters"=w356, "Simulated_CCD_Camera in"=w355) -> ("error out"=w358:errorcluster, "Simulated_CCD_Camera out"=w359:refnum<class "Simulated_CCD_Camera.lvclass">)  [unwired: 7 in]
              n171 = Bundle By Name(cluster=w366, "Simulated_CCD_Camera.lvclass"=w359) -> (w365:refnum<class "Channel.lvclass">)
            }
            frame "#SEQS" {
              n172 = Unbundle By Name(w379) -> ("Simulated_CCD_Camera.lvclass"=w374:refnum<class "Simulated_CCD_Camera.lvclass">)
              n173 = Fract/Exp String To Number(string=w375, default (0 dbl)=u32 0) -> (number=w376:u32)  [unwired: 2 in, 1 out]
              n174 = call-dynamic "Read SET parameters.vi"("error in (no error)"=w373, "Simulated_CCD_Camera in"=w374) -> ("error out"=w367:errorcluster, "New SET parameters"=w370:T3, "Simulated_CCD_Camera out"=w368:refnum<class "Simulated_CCD_Camera.lvclass">)  [unwired: 7 in]
              n175 = Bundle By Name(cluster=w370, "#SEQS"=w376) -> (w369:T3)
              n176 = call-dynamic "Write SET parameters.vi"("error in (no error)"=w367, "New SET parameters"=w369, "Simulated_CCD_Camera in"=w368) -> ("error out"=w371:errorcluster, "Simulated_CCD_Camera out"=w372:refnum<class "Simulated_CCD_Camera.lvclass">)  [unwired: 7 in]
              n177 = Bundle By Name(cluster=w379, "Simulated_CCD_Camera.lvclass"=w372) -> (w378:refnum<class "Channel.lvclass">)
            }
            frame "WAVEPLATE_POS" {
              n178 = Unbundle By Name(w393) -> ("Simulated_CCD_Camera.lvclass"=w391:refnum<class "Simulated_CCD_Camera.lvclass">)
              n179 = Decimal String To Number(string=w384) -> (number=w385:i32)  [unwired: 2 in, 1 out]
              n180 = call-dynamic "Read SET parameters.vi"("error in (no error)"=w390, "Simulated_CCD_Camera in"=w391) -> ("error out"=w386:errorcluster, "New SET parameters"=w389:T3, "Simulated_CCD_Camera out"=w387:refnum<class "Simulated_CCD_Camera.lvclass">)  [unwired: 7 in]
              n181 = Bundle By Name(cluster=w389, "WAVEPLATE_POS"=w385) -> (w388:T3)
              n182 = call-dynamic "Write SET parameters.vi"("error in (no error)"=w386, "New SET parameters"=w388, "Simulated_CCD_Camera in"=w387) -> ("error out"=w381:errorcluster, "Simulated_CCD_Camera out"=w383:refnum<class "Simulated_CCD_Camera.lvclass">)  [unwired: 7 in]
              n183 = call "process waveplate string.vi"("error in (no error)"=w381, "Simulated_CCD_Camera in"=w383) -> ("error out"=w380:errorcluster, "Simulated_CCD_Camera out"=w382:refnum<class "Simulated_CCD_Camera.lvclass">)  [unwired: 8 in]
              n184 = Bundle By Name(cluster=w393, "Simulated_CCD_Camera.lvclass"=w382) -> (w392:refnum<class "Channel.lvclass">)
            }
            frame "TEMP" {
              n185 = Unbundle By Name(w406) -> ("Simulated_CCD_Camera.lvclass"=w401:refnum<class "Simulated_CCD_Camera.lvclass">)
              n186 = Fract/Exp String To Number(string=w402, default (0 dbl)=0) -> (number=w403:i32)  [unwired: 2 in, 1 out]
              n187 = call-dynamic "Read SET parameters.vi"("error in (no error)"=w400, "Simulated_CCD_Camera in"=w401) -> ("error out"=w394:errorcluster, "New SET parameters"=w397:T3, "Simulated_CCD_Camera out"=w395:refnum<class "Simulated_CCD_Camera.lvclass">)  [unwired: 7 in]
              n188 = Bundle By Name(cluster=w397, "TEMP"=w403) -> (w396:T3)
              n189 = call-dynamic "Write SET parameters.vi"("error in (no error)"=w394, "New SET parameters"=w396, "Simulated_CCD_Camera in"=w395) -> ("error out"=w398:errorcluster, "Simulated_CCD_Camera out"=w399:refnum<class "Simulated_CCD_Camera.lvclass">)  [unwired: 7 in]
              n190 = Bundle By Name(cluster=w406, "Simulated_CCD_Camera.lvclass"=w399) -> (w405:refnum<class "Channel.lvclass">)
            }
            frame "COOLER_POWER_STATUS" {
              n191 = Unbundle By Name(w419) -> ("Simulated_CCD_Camera.lvclass"=w414:refnum<class "Simulated_CCD_Camera.lvclass">)
              n192 = Fract/Exp String To Number(string=w415, default (0 dbl)=u16 0) -> (number=w416:u16)  [unwired: 2 in, 1 out]
              n193 = call-dynamic "Read SET parameters.vi"("error in (no error)"=w413, "Simulated_CCD_Camera in"=w414) -> ("error out"=w407:errorcluster, "New SET parameters"=w410:T3, "Simulated_CCD_Camera out"=w408:refnum<class "Simulated_CCD_Camera.lvclass">)  [unwired: 7 in]
              n194 = Bundle By Name(cluster=w410, "COOLER_POWER_STATUS"=w416) -> (w409:T3)
              n195 = call-dynamic "Write SET parameters.vi"("error in (no error)"=w407, "New SET parameters"=w409, "Simulated_CCD_Camera in"=w408) -> ("error out"=w411:errorcluster, "Simulated_CCD_Camera out"=w412:refnum<class "Simulated_CCD_Camera.lvclass">)  [unwired: 7 in]
              n196 = Bundle By Name(cluster=w419, "Simulated_CCD_Camera.lvclass"=w412) -> (w418:refnum<class "Channel.lvclass">)
            }
            frame "COMMENT" {
              n197 = Unbundle By Name(w430) -> ("Simulated_CCD_Camera.lvclass"=w428:refnum<class "Simulated_CCD_Camera.lvclass">)
              n198 = call-dynamic "Read SET parameters.vi"("error in (no error)"=w427, "Simulated_CCD_Camera in"=w428) -> ("error out"=w421:errorcluster, "New SET parameters"=w424:T3, "Simulated_CCD_Camera out"=w422:refnum<class "Simulated_CCD_Camera.lvclass">)  [unwired: 7 in]
              n199 = Bundle By Name(cluster=w424, "COMMENT"=w420) -> (w423:T3)
              n200 = call-dynamic "Write SET parameters.vi"("error in (no error)"=w421, "New SET parameters"=w423, "Simulated_CCD_Camera in"=w422) -> ("error out"=w425:errorcluster, "Simulated_CCD_Camera out"=w426:refnum<class "Simulated_CCD_Camera.lvclass">)  [unwired: 7 in]
              n201 = Bundle By Name(cluster=w430, "Simulated_CCD_Camera.lvclass"=w426) -> (w429:refnum<class "Channel.lvclass">)
            }
            frame "OBSTYPE" {
              n202 = Unbundle By Name(w441) -> ("Simulated_CCD_Camera.lvclass"=w439:refnum<class "Simulated_CCD_Camera.lvclass">)
              n203 = call-dynamic "Read SET parameters.vi"("error in (no error)"=w438, "Simulated_CCD_Camera in"=w439) -> ("error out"=w432:errorcluster, "New SET parameters"=w435:T3, "Simulated_CCD_Camera out"=w433:refnum<class "Simulated_CCD_Camera.lvclass">)  [unwired: 7 in]
              n204 = Bundle By Name(cluster=w435, "OBSTYPE"=w431) -> (w434:T3)
              n205 = call-dynamic "Write SET parameters.vi"("error in (no error)"=w432, "New SET parameters"=w434, "Simulated_CCD_Camera in"=w433) -> ("error out"=w436:errorcluster, "Simulated_CCD_Camera out"=w437:refnum<class "Simulated_CCD_Camera.lvclass">)  [unwired: 7 in]
              n206 = Bundle By Name(cluster=w441, "Simulated_CCD_Camera.lvclass"=w437) -> (w440:refnum<class "Channel.lvclass">)
            }
            frame "OBJECT" {
              n207 = Unbundle By Name(w452) -> ("Simulated_CCD_Camera.lvclass"=w450:refnum<class "Simulated_CCD_Camera.lvclass">)
              n208 = call-dynamic "Read SET parameters.vi"("error in (no error)"=w449, "Simulated_CCD_Camera in"=w450) -> ("error out"=w443:errorcluster, "New SET parameters"=w446:T3, "Simulated_CCD_Camera out"=w444:refnum<class "Simulated_CCD_Camera.lvclass">)  [unwired: 7 in]
              n209 = Bundle By Name(cluster=w446, "OBJECT"=w442) -> (w445:T3)
              n210 = call-dynamic "Write SET parameters.vi"("error in (no error)"=w443, "New SET parameters"=w445, "Simulated_CCD_Camera in"=w444) -> ("error out"=w447:errorcluster, "Simulated_CCD_Camera out"=w448:refnum<class "Simulated_CCD_Camera.lvclass">)  [unwired: 7 in]
              n211 = Bundle By Name(cluster=w452, "Simulated_CCD_Camera.lvclass"=w448) -> (w451:refnum<class "Channel.lvclass">)
            }
            frame "OBSERVER" {
              n212 = Unbundle By Name(w463) -> ("Simulated_CCD_Camera.lvclass"=w461:refnum<class "Simulated_CCD_Camera.lvclass">)
              n213 = call-dynamic "Read SET parameters.vi"("error in (no error)"=w460, "Simulated_CCD_Camera in"=w461) -> ("error out"=w454:errorcluster, "New SET parameters"=w457:T3, "Simulated_CCD_Camera out"=w455:refnum<class "Simulated_CCD_Camera.lvclass">)  [unwired: 7 in]
              n214 = Bundle By Name(cluster=w457, "OBSERVER"=w453) -> (w456:T3)
              n215 = call-dynamic "Write SET parameters.vi"("error in (no error)"=w454, "New SET parameters"=w456, "Simulated_CCD_Camera in"=w455) -> ("error out"=w458:errorcluster, "Simulated_CCD_Camera out"=w459:refnum<class "Simulated_CCD_Camera.lvclass">)  [unwired: 7 in]
              n216 = Bundle By Name(cluster=w463, "Simulated_CCD_Camera.lvclass"=w459) -> (w462:refnum<class "Channel.lvclass">)
            }
            frame "FILTER" {
              n217 = Unbundle By Name(w474) -> ("Simulated_CCD_Camera.lvclass"=w472:refnum<class "Simulated_CCD_Camera.lvclass">)
              n218 = call-dynamic "Read SET parameters.vi"("error in (no error)"=w471, "Simulated_CCD_Camera in"=w472) -> ("error out"=w465:errorcluster, "New SET parameters"=w468:T3, "Simulated_CCD_Camera out"=w466:refnum<class "Simulated_CCD_Camera.lvclass">)  [unwired: 7 in]
              n219 = Bundle By Name(cluster=w468, "FILTER"=w464) -> (w467:T3)
              n220 = call-dynamic "Write SET parameters.vi"("error in (no error)"=w465, "New SET parameters"=w467, "Simulated_CCD_Camera in"=w466) -> ("error out"=w469:errorcluster, "Simulated_CCD_Camera out"=w470:refnum<class "Simulated_CCD_Camera.lvclass">)  [unwired: 7 in]
              n221 = Bundle By Name(cluster=w474, "Simulated_CCD_Camera.lvclass"=w470) -> (w473:refnum<class "Channel.lvclass">)
            }
            frame "CTRLINTE" {
              n222 = Unbundle By Name(w485) -> ("Simulated_CCD_Camera.lvclass"=w483:refnum<class "Simulated_CCD_Camera.lvclass">)
              n223 = call-dynamic "Read SET parameters.vi"("error in (no error)"=w482, "Simulated_CCD_Camera in"=w483) -> ("error out"=w476:errorcluster, "New SET parameters"=w479:T3, "Simulated_CCD_Camera out"=w477:refnum<class "Simulated_CCD_Camera.lvclass">)  [unwired: 7 in]
              n224 = Bundle By Name(cluster=w479, "CTRLINTE"=w475) -> (w478:T3)
              n225 = call-dynamic "Write SET parameters.vi"("error in (no error)"=w476, "New SET parameters"=w478, "Simulated_CCD_Camera in"=w477) -> ("error out"=w480:errorcluster, "Simulated_CCD_Camera out"=w481:refnum<class "Simulated_CCD_Camera.lvclass">)  [unwired: 7 in]
              n226 = Bundle By Name(cluster=w485, "Simulated_CCD_Camera.lvclass"=w481) -> (w484:refnum<class "Channel.lvclass">)
            }
            frame "INSTMODE" {
              n227 = Unbundle By Name(w496) -> ("Simulated_CCD_Camera.lvclass"=w494:refnum<class "Simulated_CCD_Camera.lvclass">)
              n228 = call-dynamic "Read SET parameters.vi"("error in (no error)"=w493, "Simulated_CCD_Camera in"=w494) -> ("error out"=w487:errorcluster, "New SET parameters"=w490:T3, "Simulated_CCD_Camera out"=w488:refnum<class "Simulated_CCD_Camera.lvclass">)  [unwired: 7 in]
              n229 = Bundle By Name(cluster=w490, "INSTMODE"=w486) -> (w489:T3)
              n230 = call-dynamic "Write SET parameters.vi"("error in (no error)"=w487, "New SET parameters"=w489, "Simulated_CCD_Camera in"=w488) -> ("error out"=w491:errorcluster, "Simulated_CCD_Camera out"=w492:refnum<class "Simulated_CCD_Camera.lvclass">)  [unwired: 7 in]
              n231 = Bundle By Name(cluster=w496, "Simulated_CCD_Camera.lvclass"=w492) -> (w495:refnum<class "Channel.lvclass">)
            }
            frame "TCSMODE" {
              n232 = Unbundle By Name(w509) -> ("Simulated_CCD_Camera.lvclass"=w507:refnum<class "Simulated_CCD_Camera.lvclass">)
              n233 = Equal?(x="ON", y=w498) -> (x = y?=w499:bool)
              n234 = call-dynamic "Read SET parameters.vi"("error in (no error)"=w506, "Simulated_CCD_Camera in"=w507) -> ("error out"=w500:errorcluster, "New SET parameters"=w503:T3, "Simulated_CCD_Camera out"=w501:refnum<class "Simulated_CCD_Camera.lvclass">)  [unwired: 7 in]
              n235 = Bundle By Name(cluster=w503, "TCSMODE"=w499) -> (w502:T3)
              n236 = call-dynamic "Write SET parameters.vi"("error in (no error)"=w500, "New SET parameters"=w502, "Simulated_CCD_Camera in"=w501) -> ("error out"=w504:errorcluster, "Simulated_CCD_Camera out"=w505:refnum<class "Simulated_CCD_Camera.lvclass">)  [unwired: 7 in]
              n237 = Bundle By Name(cluster=w509, "Simulated_CCD_Camera.lvclass"=w505) -> (w508:refnum<class "Channel.lvclass">)
            }
            frame "ICSMODE" {
              n238 = Unbundle By Name(w524) -> ("Simulated_CCD_Camera.lvclass"=w522:refnum<class "Simulated_CCD_Camera.lvclass">)
              n239 = Decimal String To Number(string=w516, default (0L)=u8 0 ("default (0 I32)")) -> (number=w515:u8)  [unwired: 1 in, 1 out]
              n240 = call-dynamic "Read SET parameters.vi"("error in (no error)"=w521, "Simulated_CCD_Camera in"=w522) -> ("error out"=w517:errorcluster, "New SET parameters"=w520:T3, "Simulated_CCD_Camera out"=w518:refnum<class "Simulated_CCD_Camera.lvclass">)  [unwired: 7 in]
              n241 = Bundle By Name(cluster=w520, "ICSMODE"=w515) -> (w519:T3)
              n242 = call-dynamic "Write SET parameters.vi"("error in (no error)"=w517, "New SET parameters"=w519, "Simulated_CCD_Camera in"=w518) -> ("error out"=w511:errorcluster, "Simulated_CCD_Camera out"=w513:refnum<class "Simulated_CCD_Camera.lvclass">)  [unwired: 7 in]
              n243 = call "Procces ICS mode.vi"("error in (no error)"=w511, "Simulated_CCD_Camera in"=w513) -> ("error out"=w510:errorcluster, "Simulated_CCD_Camera out"=w512:refnum<class "Simulated_CCD_Camera.lvclass">)  [unwired: 8 in]
              n244 = Bundle By Name(cluster=w524, "Simulated_CCD_Camera.lvclass"=w512) -> (w523:refnum<class "Channel.lvclass">)
            }
            frame "SUFFIX" {
              n245 = To Lower Case(string=w525) -> (all lower case string=w526:string)
              n246 = Bundle By Name(cluster=w529, "suffix of the image name"=w526) -> (w528:refnum<class "Channel.lvclass">)
            }
          }
          n247 = Unbundle By Name(w291) -> ("Simulated_CCD_Camera.lvclass"=w293:refnum<class "Simulated_CCD_Camera.lvclass">, "Image path"=w283:path, "error log file"=w282:string)
          n248 = Build Path(base path=w283, name or relative path=w282) -> (appended path=w281:path)
          n249 = call "Verify Parameters.vi"("error in (no error)"=w292, "error file"=w281, "Simulated_CCD_Camera in"=w293) -> ("error out"=w295:errorcluster, "Simulated_CCD_Camera out"=w294:refnum<class "Simulated_CCD_Camera.lvclass">)  [unwired: 7 in]
          n250 = call-dynamic "Set Camera Configuration.vi"("error in (no error)"=w295, "CCDCamera in"=w294) -> ("error out"=w284:errorcluster, "CCDCamera out"=w285:refnum<class "Simulated_CCD_Camera.lvclass">)  [unwired: 8 in]
          n251 = Bundle By Name(cluster=w291, "Simulated_CCD_Camera.lvclass"=w285) -> (w290:refnum<class "Channel.lvclass">)
          n252 = Unbundle By Name(w290) -> ("RxTx.lvclass"=w289:refnum<class "RxTx.lvclass">)
          n253 = call "Write Tx Message.vi"("error in (no error)"=w284, "Tx Message"="DONE", "RxTx in"=w289) -> ("error out"=w287:errorcluster, "RxTx out"=w288:refnum<class "RxTx.lvclass">)  [unwired: 7 in]
          n254 = call "Send TX Message.vi"("error in (no error)"=w287, "RxTx in"=w288) -> ("error out"=w307:errorcluster, "RxTx out"=w312:refnum<class "RxTx.lvclass">)  [unwired: 8 in]
          n255 = Bundle By Name(cluster=w290, "RxTx.lvclass"=w312) -> (w306:refnum<class "Channel.lvclass">)
          n256 = Unbundle By Name(w306) -> ("State Machine.lvclass"=w309:refnum<class "State Machine.lvclass">)
          n257 = call-dynamic "Write State.vi"("error in (no error)"=w307, "State"="False", "State Machine in"=w309) -> ("error out"=w304:errorcluster, "State Machine out"=w310:refnum<class "State Machine.lvclass">)  [unwired: 7 in]
          n258 = Bundle By Name(cluster=w306, "State Machine.lvclass"=w310) -> (w305:refnum<class "Channel.lvclass">)
        }
        frame "GET" {
          n259 = Unbundle By Name(w535) -> ("RxTx.lvclass"=w547:refnum<class "RxTx.lvclass">)
          n260 = call "Read Rx Value.vi"("error in (no error)"=w544, "RxTx in"=w547) -> ("error out"=w548:errorcluster, "Rx value"=w536:string)  [unwired: 7 in, 1 out]
          n261 = case shown="\"#CUBES\"" w536 {
            tunnel: [w551 w558 w565 w572 w579 w586 w588 w590 w592] -> w545
            tunnel: w535 -> [w551 w558 w565 w572 w579 w586 w588 w590 w592]
            tunnel: [w550 w553 w560 w568 w575 w582 w587 w589 w591] -> w531
            tunnel: w548 -> [w550 w552 w559 w567 w574 w581 w587 w589 w591]
            tunnel: ["INVALID_PARAMETER" w557 w564 w571 w578 w585 _ _ _] -> w530
            frame "False", Default {
            }
            frame "COOLER_POWER_STATUS" {
              n262 = Unbundle By Name(w558) -> ("Simulated_CCD_Camera.lvclass"=w555:refnum<class "Simulated_CCD_Camera.lvclass">)
              n263 = call-dynamic "Read Prev SET parameters.vi"("error in (no error)"=w552, "Simulated_CCD_Camera in"=w555) -> ("error out"=w553:errorcluster, "Old SET parameters"=w554:T3)  [unwired: 7 in, 1 out]
              n264 = Unbundle By Name(w554) -> ("COOLER_POWER_STATUS"=w556:u16)
              n265 = Number To Decimal String(number=w556) -> (decimal integer string=w557:string)  [unwired: 1 in]
            }
            frame "TEMP" {
              n266 = Unbundle By Name(w565) -> ("Simulated_CCD_Camera.lvclass"=w562:refnum<class "Simulated_CCD_Camera.lvclass">)
              n267 = call-dynamic "Read Prev SET parameters.vi"("error in (no error)"=w559, "Simulated_CCD_Camera in"=w562) -> ("error out"=w560:errorcluster, "Old SET parameters"=w561:T3)  [unwired: 7 in, 1 out]
              n268 = Unbundle By Name(w561) -> ("TEMP"=w563:i32)
              n269 = Number To Decimal String(number=w563) -> (decimal integer string=w564:string)  [unwired: 1 in]
            }
            frame "EXPTIME" {
              n270 = Unbundle By Name(w572) -> ("Simulated_CCD_Camera.lvclass"=w570:refnum<class "Simulated_CCD_Camera.lvclass">)
              n271 = call-dynamic "Read Prev SET parameters.vi"("error in (no error)"=w567, "Simulated_CCD_Camera in"=w570) -> ("error out"=w568:errorcluster, "Old SET parameters"=w569:T3)  [unwired: 7 in, 1 out]
              n272 = Unbundle By Name(w569) -> ("EXPTIME"=w566:dbl)
              n273 = Number To Fractional String(number=w566) -> (F-format string=w571:string)  [unwired: 3 in]
            }
            frame "#FRAMES" {
              n274 = Unbundle By Name(w579) -> ("Simulated_CCD_Camera.lvclass"=w577:refnum<class "Simulated_CCD_Camera.lvclass">)
              n275 = call-dynamic "Read Prev SET parameters.vi"("error in (no error)"=w574, "Simulated_CCD_Camera in"=w577) -> ("error out"=w575:errorcluster, "Old SET parameters"=w576:T3)  [unwired: 7 in, 1 out]
              n276 = Unbundle By Name(w576) -> ("#FRAMES"=w573:u32)
              n277 = Number To Decimal String(number=w573) -> (decimal integer string=w578:string)  [unwired: 1 in]
            }
            frame "#CUBES" {
              n278 = Unbundle By Name(w586) -> ("Simulated_CCD_Camera.lvclass"=w584:refnum<class "Simulated_CCD_Camera.lvclass">)
              n279 = call-dynamic "Read Prev SET parameters.vi"("error in (no error)"=w581, "Simulated_CCD_Camera in"=w584) -> ("error out"=w582:errorcluster, "Old SET parameters"=w583:T3)  [unwired: 7 in, 1 out]
              n280 = Unbundle By Name(w583) -> ("#CYCLES"=w580:u32)
              n281 = Number To Decimal String(number=w580) -> (decimal integer string=w585:string)  [unwired: 1 in]
            }
            frame "COMMENT" {
            }
            frame "SUFFIX" {
            }
            frame "OBSTYPE" {
            }
          }
          n282 = Unbundle By Name(w545) -> ("RxTx.lvclass"=w534:refnum<class "RxTx.lvclass">)
          n283 = call "Write Tx Message.vi"("error in (no error)"=w531, "Tx Message"=w530, "RxTx in"=w534) -> ("error out"=w532:errorcluster, "RxTx out"=w533:refnum<class "RxTx.lvclass">)  [unwired: 7 in]
          n284 = call "Send TX Message.vi"("error in (no error)"=w532, "RxTx in"=w533) -> ("error out"=w540:errorcluster, "RxTx out"=w546:refnum<class "RxTx.lvclass">)  [unwired: 8 in]
          n285 = Bundle By Name(cluster=w545, "RxTx.lvclass"=w546) -> (w539:refnum<class "Channel.lvclass">)
          n286 = Unbundle By Name(w539) -> ("State Machine.lvclass"=w541:refnum<class "State Machine.lvclass">)
          n287 = call-dynamic "Write State.vi"("error in (no error)"=w540, "State"="False", "State Machine in"=w541) -> ("error out"=w537:errorcluster, "State Machine out"=w543:refnum<class "State Machine.lvclass">)  [unwired: 7 in]
          n288 = Bundle By Name(cluster=w539, "State Machine.lvclass"=w543) -> (w538:refnum<class "Channel.lvclass">)
        }
        frame "RESTART_COMMUNICATION" {
          n289 = Unbundle By Name(w603) -> ("Simulated_CCD_Camera.lvclass"=w598:refnum<class "Simulated_CCD_Camera.lvclass">, "Channel ID"=w593:u8)
          n290 = call-dynamic "Initialize Camera.vi"("error in (no error)"=w604, "channel"=w593, "CCDCamera in"=w598) -> ("error out"=w601:errorcluster, "CCDCamera out"=w597:refnum<class "Simulated_CCD_Camera.lvclass">)  [unwired: 6 in, 1 out]
          n291 = Bundle By Name(cluster=w603, "Simulated_CCD_Camera.lvclass"=w597) -> (w599:refnum<class "Channel.lvclass">)
          n292 = Unbundle By Name(w599) -> ("State Machine.lvclass"=w600:refnum<class "State Machine.lvclass">)
          n293 = call-dynamic "Write State.vi"("error in (no error)"=w601, "State"="False", "State Machine in"=w600) -> ("error out"=w595:errorcluster, "State Machine out"=w596:refnum<class "State Machine.lvclass">)  [unwired: 7 in]
          n294 = Bundle By Name(cluster=w599, "State Machine.lvclass"=w596) -> (w602:refnum<class "Channel.lvclass">)
        }
        frame "WAIT_RECONNECTION" {
          n295 = Unbundle By Name(w610) -> ("State Machine.lvclass"=w614:refnum<class "State Machine.lvclass">)
          n296 = call "Verify Timer.vi"("error in (no error)"=w613, "State Machine in"=w614) -> ("error out"=w611:errorcluster, "time out"=w608:bool, "State Machine out"=w612:refnum<class "State Machine.lvclass">)  [unwired: 7 in]
          n297 = case shown="True" w608 {
            tunnel: ["WAIT_RECONNECTION" "RESTART_COMMUNICATION"] -> w607
            frame False {
            }
            frame True {
            }
          }
          n298 = call-dynamic "Write State.vi"("error in (no error)"=w611, "State"=w607, "State Machine in"=w612) -> ("error out"=w605:errorcluster, "State Machine out"=w609:refnum<class "State Machine.lvclass">)  [unwired: 7 in]
          n299 = Bundle By Name(cluster=w610, "State Machine.lvclass"=w609) -> (w606:refnum<class "Channel.lvclass">)
        }
      }
    }
    frame Error {
    }
  }
  "error out" <- w3
  "Channel out" <- w1
